vi "流程固件设置对话框.vi"() -> ()   [LabVIEW 2016, in "斯坦道总氮.lvlib"]
uses:
  <vilib>/Utility/miscctls.llb/LVPointTypeDef.ctl
panel:
  in  "关闭":bool
  in  "外设设置":bool
  in  "固件升级":bool
  in  "流程写入":bool
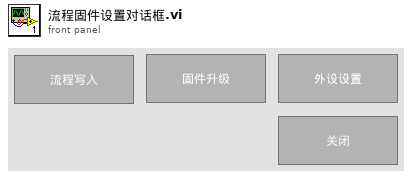
[diagram p1: front panel]
types:
  T1 = typedef "LVPointTypeDef.ctl" = cluster{"Horizontal":i16, "Vertical":i16}
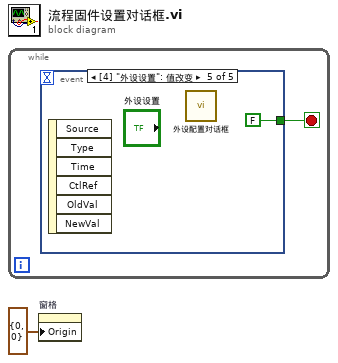
[diagram p0: block diagram]
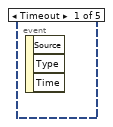
[diagram p2: hidden frame]
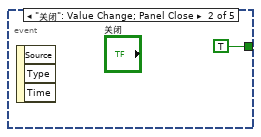
[diagram p3: hidden frame]
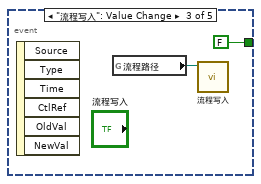
[diagram p4: hidden frame]
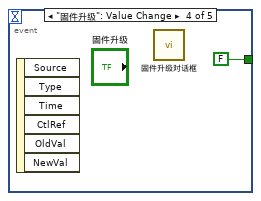
[diagram p5: hidden frame]
diagram:
  n1 = while {
    stop <- w2 stop-if-true
    n2 = event shown="[4] \"外设设置\": 值改变" {
      selector: _ -> [_ _ _ _ _]
      dyn-events: _ -> [_ _ _ _ _]
      timeout: _ -> [_ _ _ _ _]
      tunnel: [_ TRUE FALSE FALSE FALSE] -> w2
      event Timeout {
        n3 = event-data() -> ()  [unwired: 1 in, 3 out]
      }
      event "关闭": Value Change; Panel Close {
        n4 = event-data() -> ()  [unwired: 1 in, 3 out]
      }
      event "流程写入": Value Change {
        n5 = event-data() -> ()  [unwired: 1 in, 6 out]
        n6 = global read "总磷总氮断电保存全局变量.vi" "流程路径"() -> (w4:path)
        n7 = call "流程写入.vi"("添加的路径"=w4) -> ()  [unwired: 11 in]
      }
      event "固件升级": Value Change {
        n8 = event-data() -> ()  [unwired: 1 in, 6 out]
        n9 = call "固件升级对话框.vi"() -> ()  [unwired: 12 in]
      }
      event "外设设置": Value Change {
        n10 = event-data() -> ()  [unwired: 1 in, 6 out]
        n11 = call "外设配置对话框.vi"() -> ()  [unwired: 12 in]
      }
    }
  }
  n12 = property on="窗格" class="Pane"("Origin"=T1 {"Horizontal"=0, "Vertical"=0} ("原点")) -> ()  [unwired: 2 in, 2 out]
